vi "GUI_Main.vi"() -> ()   [LabVIEW 2020]
panel:
  out "Sampling Rate":dbl
  out "No. of Channels":dbl
  out "No. of Bits":dbl
  in  "Exit":bool
  in  "ADC Type":enum16{""}(ring)
  in  "Channel":enum16{""}(ring)
  in  "OK":bool
  in  "File Path":path
  out "Digital Waveform":T1(graph)
  in  "Start Btn":bool
  in  "Stop Btn":bool
  # "MULTICHANNEL ADC"
  # "SOLITON"
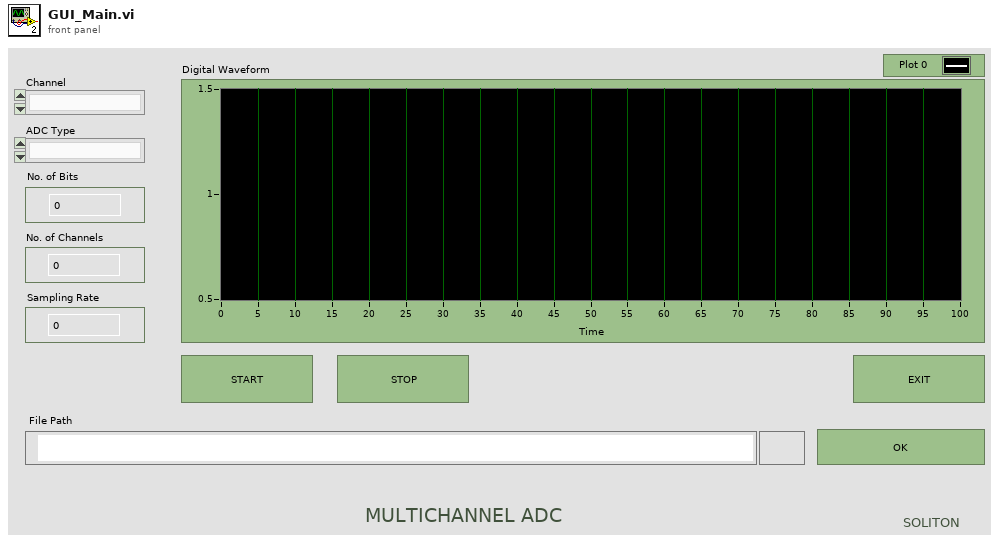
[diagram p1: front panel]
types:
  T1 = cluster{"x0":dbl, "dx":dbl, "[y]":u8[], "ports":i32}
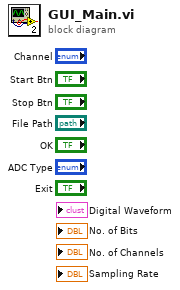
[diagram p0: block diagram]
diagram:
